vi "Time.SQL DateTime String to TimeStamp.vi"(11 "Time String In":string) -> (3 "Time Stamp Out":timestamp)   [LabVIEW 2019]
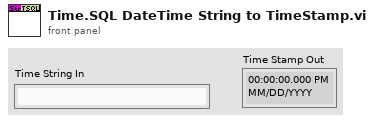
[diagram p1: front panel]
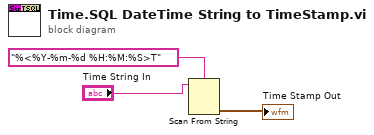
[diagram p0: block diagram]
diagram:
  n1 = Scan From String(format string="%<%Y-%m-%d %H:%M:%S>T", input string="Time String In") -> (output 1=→"Time Stamp Out":timestamp)  [unwired: 3 in, 3 out]
